vi "WSVCAP SHL Host LL I2C Build and Parse Write Message.vi"(0 "C Write Data In [DUT Ordered]":u8[][](array[numeric]) format="%.0x", 4 "Socket Mask [U64] In":u64=1 format="%016x", 5 "error in":errorcluster, 6 "Message In":string, 7 "Sub Address In":u8=20 format="%.0x") -> (11 "UUT Set (0/1) Out (Legacy)":u8=20 format="%.0x", 12 "Message Out":string, 13 "Sub Address Out":u8=20 format="%.0x", 14 "C Write Data Out [DUT Ordered]":u8[][](array[numeric]) format="%.0x", 18 "Socket Mask [U64] Out":u64=1 format="%08x", 19 "error out":errorcluster)   [LabVIEW 2017]
panel:
  in  "UUT Set (0/1) In (Legacy)":u8 format="%.0x"
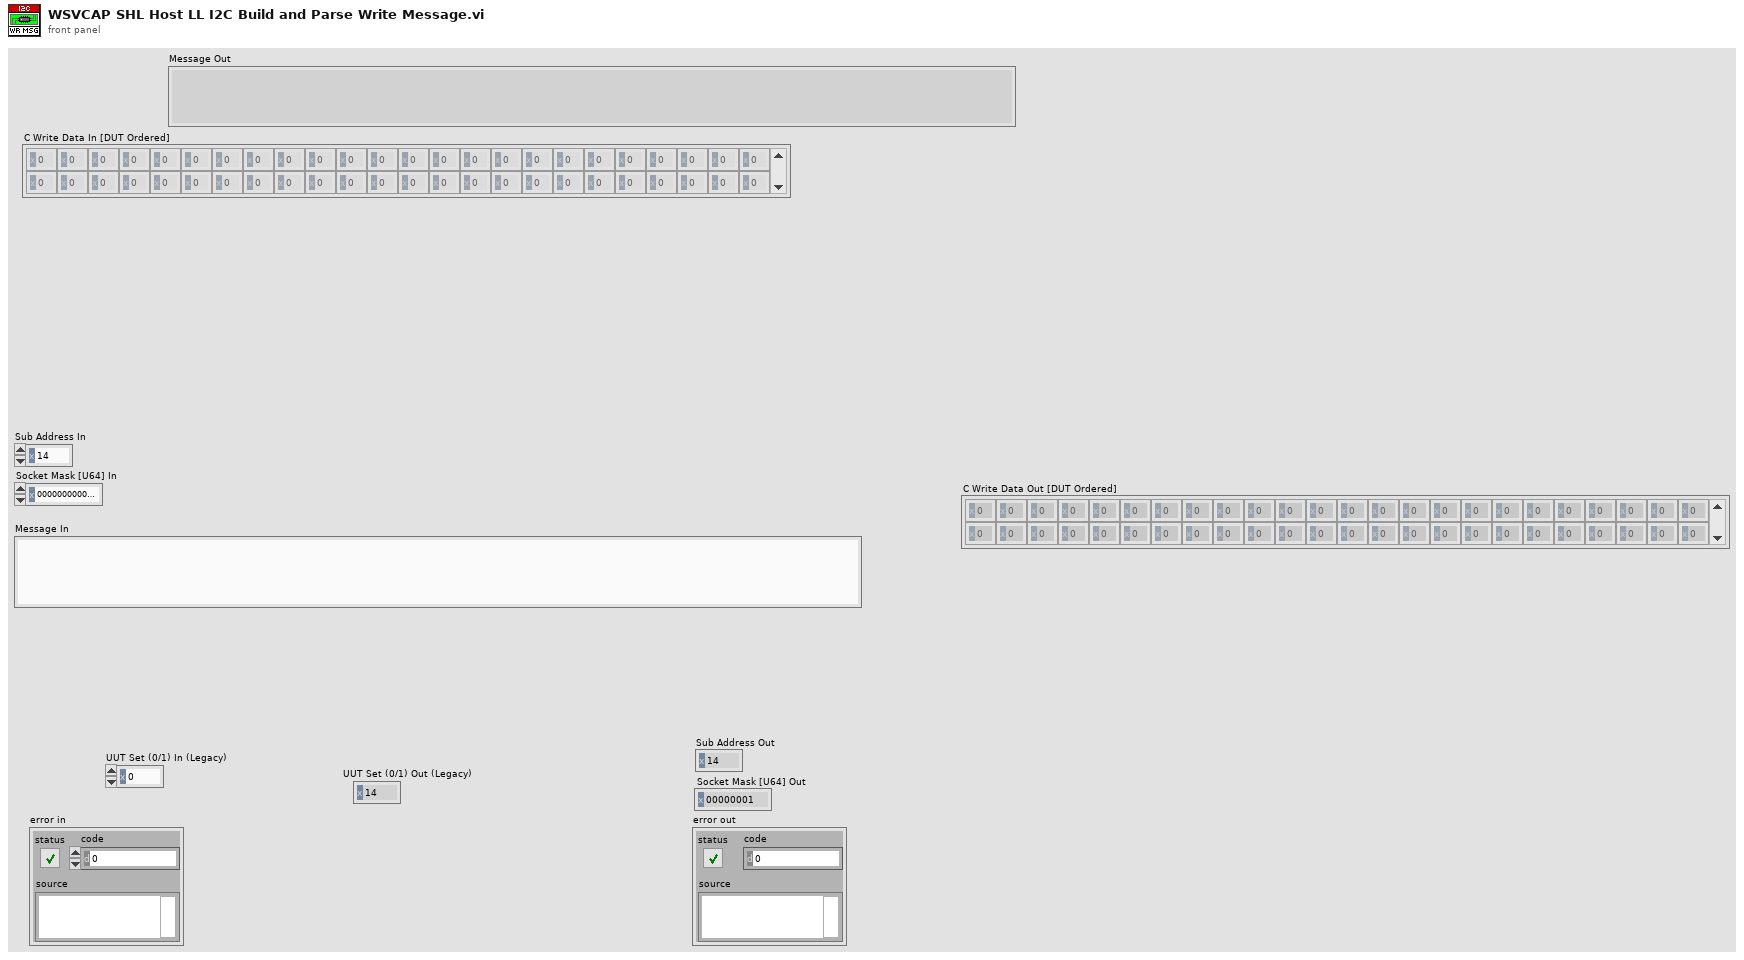
[diagram p1: front panel]
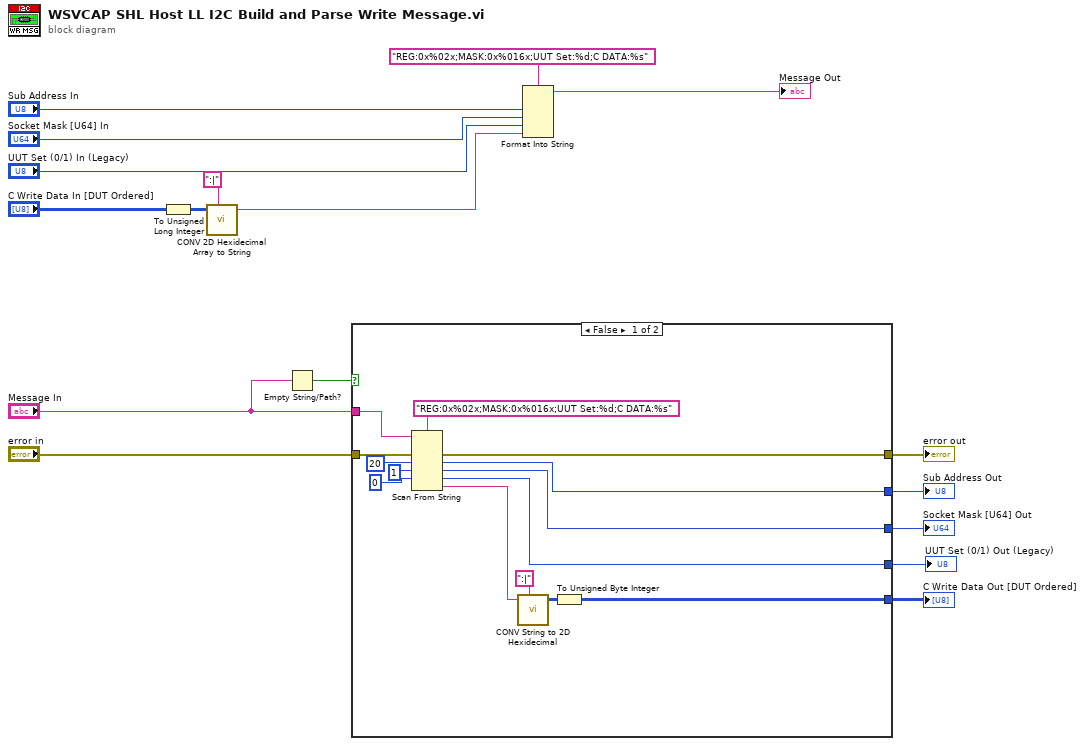
[diagram p0: block diagram]
diagram:
  n1 = To Unsigned Long Integer(number="C Write Data In [DUT Ordered]") -> (unsigned 32bit integer=w17:u32[][])
  n2 = call "CONV 2D Hexidecimal Array to String.vi"("2-D Hexidecimal"=w17, "Delimiters (,;)"=":|") -> ("String"=w14:string)  [unwired: 7 in]
  n3 = Empty String/Path?(string/path="Message In") -> (empty?=w5:bool)
  n4 = case shown="False" w5 {
    tunnel: [w30 _] -> w12
    tunnel: [w28 _] -> w11
    tunnel: [w27 _] -> w10
    tunnel: "error in" -> [w25 w32]
    tunnel: [w24 w32] -> w7
    tunnel: "Message In" -> [w23 _]
    tunnel: [w19 _] -> w3
    frame False {
      n5 = Scan From String(format string="REG:0x%02x;MASK:0x%016x;UUT Set:%d;C DATA:%s", input string=w23, error in=w25, default 1=u8 20 ("Sub Address Out"), default 2=u64 1 ("Socket Mask [U32] Out"), default 3=u8 0 ("Sub Address Out")) -> (error out=w24:errorcluster, output 1=w28:u8, output 2=w27:u64, output 3=w19:u8, output 4=w26:string)  [unwired: 2 in, 2 out]
      n6 = call "CONV String to 2D Hexidecimal.vi"("String"=w26, "Delimiters (,;)"=":|") -> ("2-D Hexidecimal"=w31:u32[][])  [unwired: 7 in]
      n7 = To Unsigned Byte Integer(number=w31) -> (unsigned 8bit integer=w30:u8[][])
    }
    frame True {
    }
  }
  "C Write Data Out [DUT Ordered]" <- w12
  "Sub Address Out" <- w11
  "Socket Mask [U64] Out" <- w10
  "error out" <- w7
  "UUT Set (0/1) Out (Legacy)" <- w3
  n8 = Format Into String(format string="REG:0x%02x;MASK:0x%016x;UUT Set:%d;C DATA:%s", "Sub Address In", "Socket Mask [U64] In", "UUT Set (0/1) In (Legacy)", w14) -> (resulting string=→"Message Out":string)  [unwired: 2 in, 1 out]
